vi "StartProcess.vi"(7 "型号":enum16{"长安", "江淮"}(ring), 8 "error in":errorcluster caption="错误输入（无错误）", 9 "延时":i32=100, 10 "Cycles":i32=5, 11 "COMIn":refnum<visa-resource-name>) -> (0 "error out":errorcluster caption="错误输出", 1 "连接的字符串":string, 2 "Time":u32, 3 "OK？":bool)   [LabVIEW 2013]
uses:
  <vilib>/Instr/_visa.llb/VISA Flush IO Buffer Mask.ctl
  <vilib>/Instr/_visa.llb/VISA Configure Serial Port (Instr).vi
panel:
  out "数组 2":string[](array[string])
  out "数组":string[](array[string])
  out "读取缓冲区 3":string
  out "字符串 2":string
  out "读取缓冲区 2":string
  out "字符串":string
  in  "CMD":enum16{"启动进程", "退出进程"}(ring)
  out "读取缓冲区":string
  # "长安登录与启动localdata：\n用户名：root\n密码：quectel123\n启动localdata：/data/QuecOpen/local_data\n江淮登录与启动localdata：\n用户名：root\n密码：oelinux_ls123\n启动localdata：/vendor/app/local_data\n启动localdata修改为：/vendor/app/auto_test_main"
  # "延时取100时较为稳定"
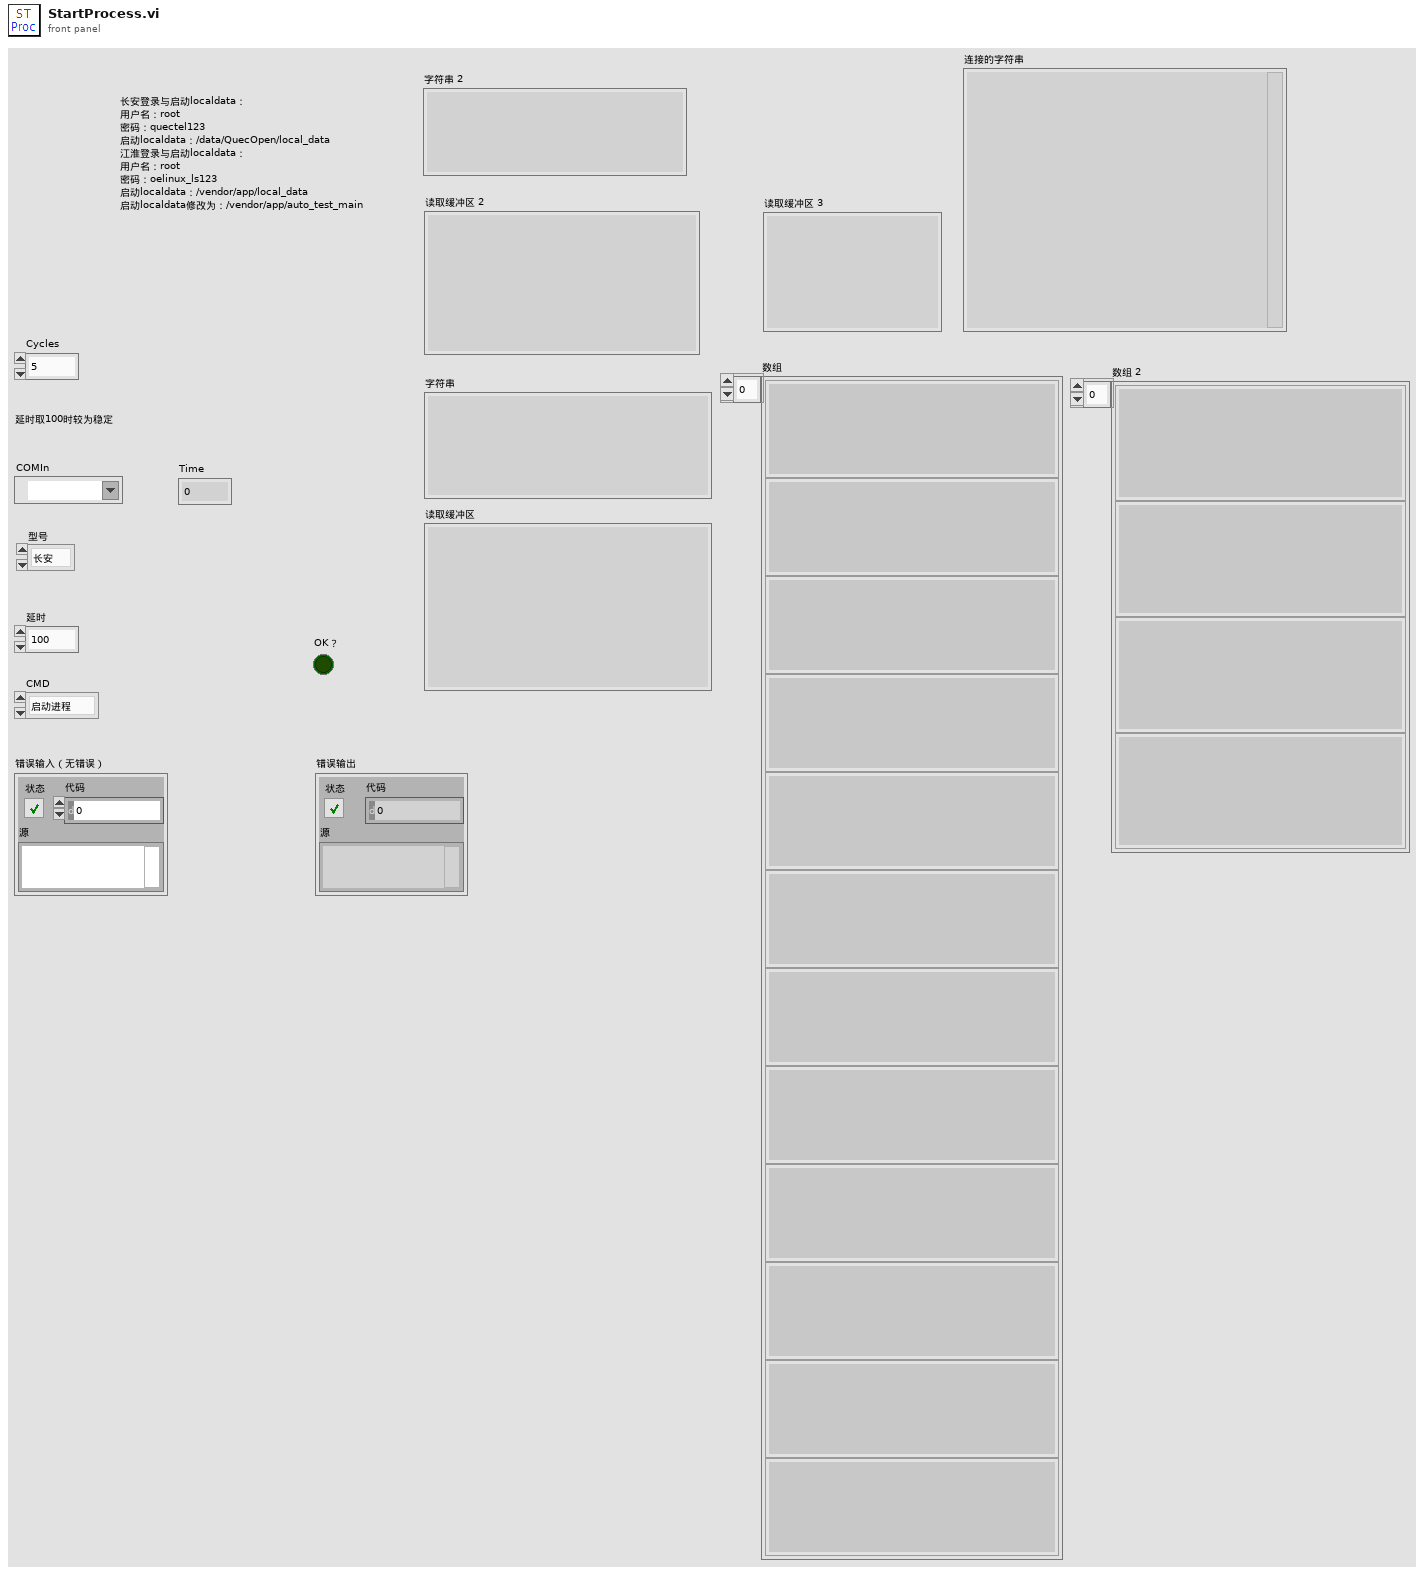
[diagram p1: front panel]
types:
  T1 = typedef "VISA Flush IO Buffer Mask.ctl" = u16
  T2 = cluster{"波特率":u32, "数据比特":u16, "奇偶":enum16{"None", "Odd", "Even", "Mark", "Space"}, "停止位":u16, "流控制":u16}
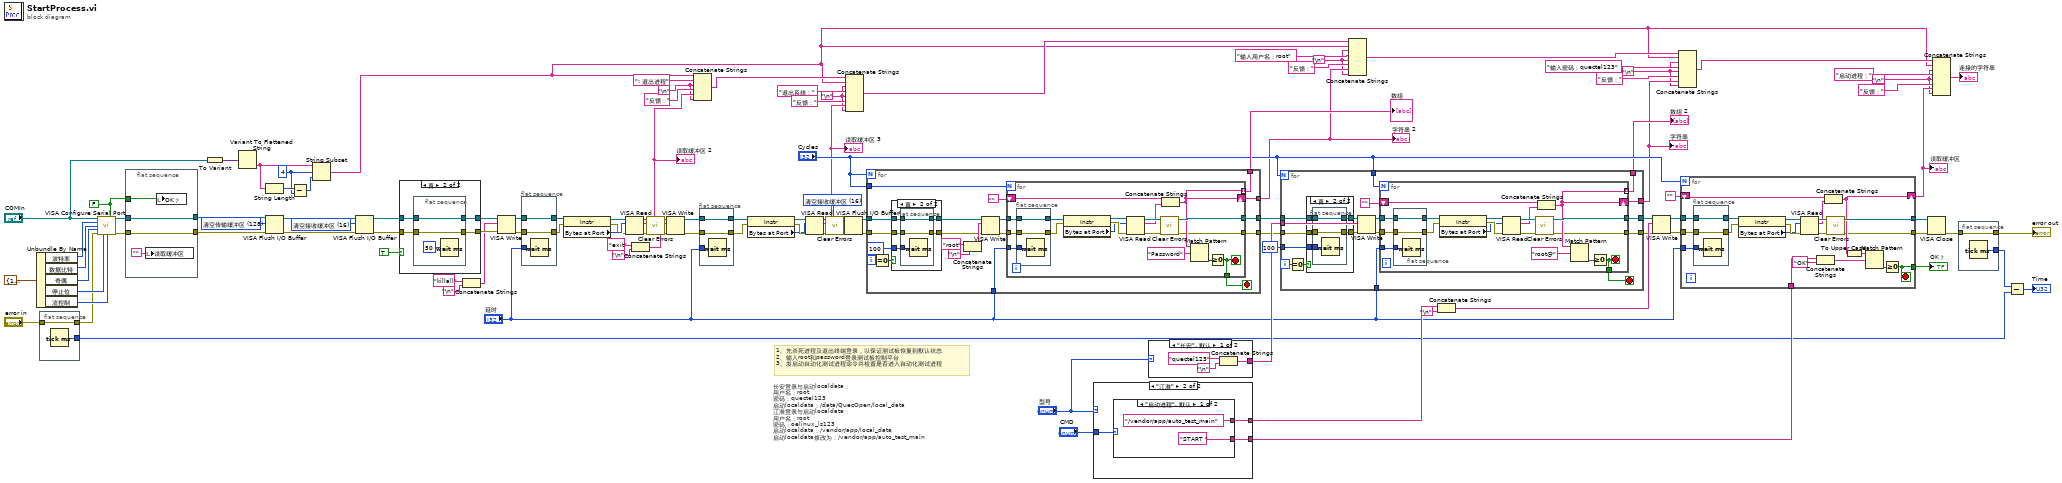
[diagram p0: block diagram]
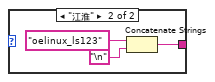
[diagram p2: hidden frame]
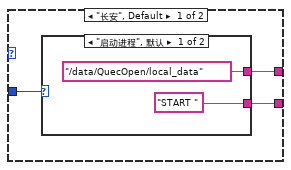
[diagram p3: hidden frame]
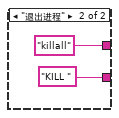
[diagram p4: hidden frame]
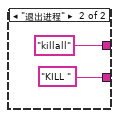
[diagram p5: hidden frame]
diagram:
  w3 = "\n"
  w6 = "\n"
  w8 = "\n"
  w10 = "\n"
  w25 = "\n"
  w31 = 4 ("偏移量(0)")
  w57 = T1 16 items=["清空接收缓冲区"=16, "向设备写入传输缓冲区"=32, "清空接收缓冲区（无I/O）"=64, "清空传输缓冲区"=128] ("Mask")
  w103 = T1 16 items=["清空接收缓冲区"=16, "向设备写入传输缓冲区"=32, "清空接收缓冲区（无I/O）"=64, "清空传输缓冲区"=128] ("Mask")
  w104 = T1 128 items=["清空接收缓冲区"=16, "向设备写入传输缓冲区"=32, "清空接收缓冲区（无I/O）"=64, "清空传输缓冲区"=128] ("Mask")
  w1 = FALSE ("Enable Termination\nChar (T)")
  # "长安登录与启动localdata：\n用户名：root\n密码：quectel123\n启动localdata：/data/QuecOpen/local_data\n江淮登录与启动localdata：\n用户名：root\n密码：oelinux_ls123\n启动localdata：/vendor/app/local_data\n启动localdata修改为：/vendor/app/auto_test_main"
  # "1、先杀死进程及退出终端登录，以保证测试板恢复到默认状态\n2、输入root和password登录测试板控制平台\n3、发启动自动化测试进程命令并检查是否进入自动化测试进程"
  n1 = Unbundle By Name(T2 {"波特率"=115200, "数据比特"=8, "奇偶"=enum."None", "停止位"=10, "流控制"=0} ("串口设置")) -> ("波特率"=w109:u32, "数据比特"=w108:u16, "奇偶"=w107:enum16{"None", "Odd", "Even", "Mark", "Space"}, "停止位"=w106:u16, "流控制"=w105:u16)
  n2 = flat-sequence {
    tunnel: [w112] -> w47
    tunnel: "error in" -> [w112]
    tunnel: [w111] -> w42
    frame #0 {
      n3 = Tick Count (ms)() -> (millisecond timer value=w111:u32)
    }
  }
  n4 = call-poly "VISA Configure Serial Port"("VISA resource name"="COMIn", "Enable Termination\nChar (T)"=w1, "baud rate (9600)"=w109, "data bits (8)"=w108, "parity (0:none)"=w107, "error in (no error)"=w47, "stop bits (10: 1 bit)"=w106, "flow control (0:none)"=w105) -> ("VISA resource name out"=w91:refnum<visa-resource-name>, "error out"=w92:errorcluster)  [unwired: 6 in]
  n5 = flat-sequence {
    tunnel: [w116] -> w93
    tunnel: w92 -> [w116]
    tunnel: [w114] -> w90
    tunnel: w91 -> [w114]
    tunnel: w1 -> [w113]
    frame #0 {
      n6 = local write "读取缓冲区"("") -> ()
      n7 = local write "OK？"(w113) -> ()
    }
  }
  n8 = To Variant(anything="COMIn") -> (Variant=w34:variant)
  n9 = Variant To Flattened String(Variant=w34) -> (data string=w33:string)  [unwired: 1 out]
  n10 = String Length(string=w33) -> (length=w32:i32)
  n11 = VISA Flush I/O Buffer(VISA resource name=w90, mask (16)=w104, error in (no error)=w93) -> (VISA resource name out=w102:refnum<visa-resource-name>, error out=w101:errorcluster)
  n12 = Subtract(x=w32, y=w31) -> (x-y=w30:i32)
  n13 = String Subset(string=w33, offset (0)=w31, length (rest)=w30) -> (substring=w4:string)
  n14 = VISA Flush I/O Buffer(VISA resource name=w102, mask (16)=w103, error in (no error)=w101) -> (VISA resource name out=w100:refnum<visa-resource-name>, error out=w99:errorcluster)
  n15 = case shown="真" TRUE {
    tunnel: w100 -> [w118 w122]
    tunnel: w99 -> [w117 w119]
    tunnel: [w118 w121] -> w82
    tunnel: [w117 w120] -> w81
    frame False {
    }
    frame True {
      n16 = flat-sequence {
        tunnel: [w124] -> w121
        tunnel: w122 -> [w124]
        tunnel: [w123] -> w120
        tunnel: w119 -> [w123]
        frame #0 {
          n17 = Wait (ms)(milliseconds to wait=u32 50 ("毫秒倍数")) -> ()  [unwired: 1 out]
        }
      }
    }
  }
  n18 = Concatenate Strings("killall" ("CMD 2"), "\n") -> (w78:string)
  n19 = VISA Write(VISA resource name=w82, write buffer=w78, error in (no error)=w81) -> (VISA resource name out=w83:refnum<visa-resource-name>, error out=w84:errorcluster)  [unwired: 1 out]
  n20 = flat-sequence {
    tunnel: [w128] -> w85
    tunnel: w83 -> [w128]
    tunnel: [w127] -> w86
    tunnel: w84 -> [w127]
    tunnel: "延时" -> [w126]
    frame #0 {
      n21 = Wait (ms)(milliseconds to wait=w126) -> ()  [unwired: 1 out]
    }
  }
  n22 = property class="Instr"(reference=w85, error in=w86) -> (reference out=w89:refnum<visa-resource-name>, error out=w87:errorcluster, "Bytes at Port"=w88:u32)
  n23 = VISA Read(VISA resource name=w89, byte count=w88, error in (no error)=w87) -> (VISA resource name out=w67:refnum<visa-resource-name>, read buffer=w26:string, error out=w66:errorcluster)  [unwired: 1 out]
  "读取缓冲区 2" <- w26
  n24 = Concatenate Strings("exit" ("CMD 2"), "\n") -> (w63:string)
  n25 = call <vilib>:"Clear Errors.vi"("error in (no error)"=w66) -> ("error out"=w36:errorcluster)  [unwired: 6 in]
  n26 = VISA Write(VISA resource name=w67, write buffer=w63, error in (no error)=w36) -> (VISA resource name out=w62:refnum<visa-resource-name>, error out=w61:errorcluster)  [unwired: 1 out]
  n27 = Concatenate Strings(w4, ": 退出进程", w25, "反馈：", w26, w25) -> (w11:string)
  n28 = flat-sequence {
    tunnel: [w131] -> w53
    tunnel: w62 -> [w131]
    tunnel: [w130] -> w52
    tunnel: w61 -> [w130]
    tunnel: "延时" -> [w129]
    frame #0 {
      n29 = Wait (ms)(milliseconds to wait=w129) -> ()  [unwired: 1 out]
    }
  }
  n30 = property class="Instr"(reference=w53, error in=w52) -> (reference out=w54:refnum<visa-resource-name>, error out=w56:errorcluster, "Bytes at Port"=w55:u32)
  n31 = VISA Read(VISA resource name=w54, byte count=w55, error in (no error)=w56) -> (VISA resource name out=w51:refnum<visa-resource-name>, read buffer=w22:string, error out=w50:errorcluster)  [unwired: 1 out]
  "读取缓冲区 3" <- w22
  n32 = call <vilib>:"Clear Errors.vi"("error in (no error)"=w50) -> ("error out"=w35:errorcluster)  [unwired: 6 in]
  n33 = VISA Flush I/O Buffer(VISA resource name=w51, mask (16)=w57, error in (no error)=w35) -> (VISA resource name out=w59:refnum<visa-resource-name>, error out=w58:errorcluster)
  n34 = Concatenate Strings(w11, w4, w10, "退出系统：", w10, "反馈：", w22, w10) -> (w9:string)
  n35 = for {
    N: "Cycles" -> [_]
    tunnel: [w146] -> w71
    tunnel: [w145] -> w40
    tunnel: w59 -> [w139]
    tunnel: w58 -> [w138]
    tunnel: "延时" -> [w132]
    tunnel: "Cycles" -> [w142]
    tunnel: [w141] -> w19
    tunnel: [w135] -> w49
    i -> [w134]
    stop <- w143 stop-if-true
    n36 = Equal To 0?(x=w134) -> (x = 0?=w133:bool)
    n37 = case shown="真" w133 {
      tunnel: [w153 w158] -> w140
      tunnel: w139 -> [w153 w157]
      tunnel: w138 -> [w152 w156]
      tunnel: [w152 w155] -> w137
      tunnel: 100 -> [_ w154]
      frame False {
      }
      frame True {
        n38 = flat-sequence {
          tunnel: [w161] -> w158
          tunnel: w157 -> [w161]
          tunnel: [w160] -> w155
          tunnel: w156 -> [w160]
          tunnel: [w159] -> _
          tunnel: w154 -> [w159]
          frame #0 {
            n39 = Wait (ms)(milliseconds to wait=w159) -> ()  [unwired: 1 out]
          }
        }
      }
    }
    n40 = Concatenate Strings("root", "\n") -> (w148:string)
    n41 = VISA Write(VISA resource name=w140, write buffer=w148, error in (no error)=w137) -> (VISA resource name out=w147:refnum<visa-resource-name>, error out=w151:errorcluster)  [unwired: 1 out]
    n42 = for {
      N: w142 -> [_]
      tunnel: w151 -> [w178]
      tunnel: w147 -> [w177]
      tunnel: [w176] -> w146
      tunnel: [w162] -> w145
      tunnel: w132 -> [w166]
      shift-right: [w163] -> w141
      shift-left: "" -> [w165]
      tunnel: [w164] -> w143
      tunnel: [w163] -> w135 mode=indexing
      stop <- w164 stop-if-true
      n43 = flat-sequence {
        tunnel: [w181] -> w174
        tunnel: w177 -> [w181]
        tunnel: [w180] -> w173
        tunnel: w178 -> [w180]
        tunnel: w166 -> [w179]
        frame #0 {
          n44 = Wait (ms)(milliseconds to wait=w179) -> ()  [unwired: 1 out]
        }
      }
      n45 = property class="Instr"(reference=w174, error in=w173) -> (reference out=w170:refnum<visa-resource-name>, error out=w172:errorcluster, "Bytes at Port"=w171:u32)
      n46 = VISA Read(VISA resource name=w170, byte count=w171, error in (no error)=w172) -> (VISA resource name out=w176:refnum<visa-resource-name>, read buffer=w169:string, error out=w175:errorcluster)  [unwired: 1 out]
      n47 = call <vilib>:"Clear Errors.vi"("error in (no error)"=w175) -> ("error out"=w162:errorcluster)  [unwired: 6 in]
      n48 = Concatenate Strings(w165, w169) -> (w163:string)
      n49 = Match Pattern(string=w163, regular expression="Password") -> (offset past match=w168:i32)  [unwired: 1 in, 3 out]
      n50 = Greater Or Equal To 0?(x=w168) -> (x >= 0?=w164:bool)
    }
  }
  "字符串 2" <- w19
  "数组" <- w49
  n51 = case shown="\"江淮\"" "型号" {
    tunnel: "CMD" -> [w184 w191]
    tunnel: [w183 w190] -> w73
    tunnel: [w182 w189] -> w72
    frame "长安", Default {
      n52 = case shown="\"启动进程\", 默认" w184 {
        tunnel: ["/data/QuecOpen/local_data" ("CMD 2") "killall" ("CMD 2")] -> w183
        tunnel: ["START " ("CMD 2") "KILL " ("CMD 2")] -> w182
        frame "启动进程", Default {
        }
        frame "退出进程" {
        }
      }
    }
    frame "江淮" {
      n53 = case shown="\"启动进程\", 默认" w191 {
        tunnel: ["/vendor/app/auto_test_main" ("CMD 2") "killall" ("CMD 2")] -> w190
        tunnel: ["START " ("CMD 2") "KILL " ("CMD 2")] -> w189
        frame "启动进程", Default {
        }
        frame "退出进程" {
        }
      }
    }
  }
  n54 = case shown="\"长安\", 默认" "型号" {
    tunnel: [w196 w199] -> w70
    frame "长安", Default {
      n55 = Concatenate Strings("quectel123", "\n") -> (w196:string)
    }
    frame "江淮" {
      n56 = Concatenate Strings("oelinux_ls123", "\n") -> (w199:string)
    }
  }
  n57 = for {
    N: "Cycles" -> [_]
    tunnel: w71 -> [w209]
    tunnel: w70 -> [w219]
    tunnel: [w217] -> w69
    tunnel: [w215] -> w68
    tunnel: [w214] -> w16
    tunnel: "延时" -> [w213]
    tunnel: "Cycles" -> [w211]
    tunnel: w40 -> [w207]
    tunnel: 100 -> [w205]
    tunnel: [w204] -> w37
    i -> [w203]
    stop <- w210 stop-if-true
    n58 = Equal To 0?(x=w203) -> (x = 0?=w202:bool)
    n59 = case shown="真" w202 {
      tunnel: w209 -> [w221 w226]
      tunnel: [w221 w225] -> w208
      tunnel: w207 -> [w220 w224]
      tunnel: [w220 w223] -> w206
      tunnel: w205 -> [_ w222]
      frame False {
      }
      frame True {
        n60 = flat-sequence {
          tunnel: [w229] -> w225
          tunnel: w226 -> [w229]
          tunnel: [w228] -> w223
          tunnel: w224 -> [w228]
          tunnel: [w227] -> _
          tunnel: w222 -> [w227]
          frame #0 {
            n61 = Wait (ms)(milliseconds to wait=w227) -> ()  [unwired: 1 out]
          }
        }
      }
    }
    n62 = VISA Write(VISA resource name=w208, write buffer=w219, error in (no error)=w206) -> (VISA resource name out=w218:refnum<visa-resource-name>, error out=w216:errorcluster)  [unwired: 1 out]
    n63 = for {
      N: w211 -> [_]
      tunnel: w216 -> [w246]
      tunnel: w213 -> [w245]
      tunnel: w218 -> [w244]
      tunnel: [w238] -> w217
      tunnel: [w230] -> w215
      shift-right: [w231] -> w214
      shift-left: "" -> [w236]
      tunnel: [w232] -> w210
      tunnel: [w231] -> w204 mode=indexing
      stop <- w232 stop-if-true
      n64 = flat-sequence {
        tunnel: [w249] -> w243
        tunnel: w244 -> [w249]
        tunnel: [w248] -> w242
        tunnel: w246 -> [w248]
        tunnel: w245 -> [w247]
        frame #0 {
          n65 = Wait (ms)(milliseconds to wait=w247) -> ()  [unwired: 1 out]
        }
      }
      n66 = property class="Instr"(reference=w243, error in=w242) -> (reference out=w239:refnum<visa-resource-name>, error out=w241:errorcluster, "Bytes at Port"=w240:u32)
      n67 = VISA Read(VISA resource name=w239, byte count=w240, error in (no error)=w241) -> (VISA resource name out=w238:refnum<visa-resource-name>, read buffer=w235:string, error out=w237:errorcluster)  [unwired: 1 out]
      n68 = call <vilib>:"Clear Errors.vi"("error in (no error)"=w237) -> ("error out"=w230:errorcluster)  [unwired: 6 in]
      n69 = Concatenate Strings(w236, w235) -> (w231:string)
      n70 = Match Pattern(string=w231, regular expression="root@") -> (offset past match=w234:i32)  [unwired: 1 in, 3 out]
      n71 = Greater Or Equal To 0?(x=w234) -> (x >= 0?=w232:bool)
    }
  }
  "字符串" <- w16
  "数组 2" <- w37
  n72 = Concatenate Strings(w9, w4, w8, "输入用户名：root", w8, "反馈：", w19, w8) -> (w7:string)
  n73 = Concatenate Strings(w73, "\n") -> (w76:string)
  n74 = VISA Write(VISA resource name=w69, write buffer=w76, error in (no error)=w68) -> (VISA resource name out=w75:refnum<visa-resource-name>, error out=w74:errorcluster)  [unwired: 1 out]
  n75 = Concatenate Strings(w7, w4, w6, "输入密码：quectel123", w6, "反馈：", w16, w6) -> (w5:string)
  n76 = for {
    N: "Cycles" -> [_]
    tunnel: [w269] -> w97
    tunnel: [w250] -> w96
    tunnel: [w251] -> w95
    tunnel: w75 -> [w267]
    tunnel: w74 -> [w266]
    tunnel: w72 -> [w257]
    tunnel: "延时" -> [w255]
    shift-right: [w252] -> w13
    shift-left: "" -> [w254]
    stop <- w251 stop-if-true
    n77 = flat-sequence {
      tunnel: [w272] -> w265
      tunnel: w267 -> [w272]
      tunnel: [w271] -> w264
      tunnel: w266 -> [w271]
      tunnel: w255 -> [w270]
      frame #0 {
        n78 = Wait (ms)(milliseconds to wait=w270) -> ()  [unwired: 1 out]
      }
    }
    n79 = property class="Instr"(reference=w265, error in=w264) -> (reference out=w261:refnum<visa-resource-name>, error out=w263:errorcluster, "Bytes at Port"=w262:u32)
    n80 = VISA Read(VISA resource name=w261, byte count=w262, error in (no error)=w263) -> (VISA resource name out=w269:refnum<visa-resource-name>, read buffer=w253:string, error out=w268:errorcluster)  [unwired: 1 out]
    n81 = Concatenate Strings(w257, "OK" ("正则表达式")) -> (w256:string)
    n82 = Concatenate Strings(w254, w253) -> (w252:string)
    n83 = call <vilib>:"Clear Errors.vi"("error in (no error)"=w268) -> ("error out"=w250:errorcluster)  [unwired: 6 in]
    n84 = To Upper Case(1:w252) -> (0:w259:string)
    n85 = Match Pattern(string=w259, regular expression=w256) -> (offset past match=w260:i32)  [unwired: 1 in, 3 out]
    n86 = Greater Or Equal To 0?(x=w260) -> (x >= 0?=w251:bool)
  }
  "OK？" <- w95
  "读取缓冲区" <- w13
  n87 = VISA Close(VISA resource name=w97, error in (no error)=w96) -> (error out=w45:errorcluster)
  n88 = Concatenate Strings(w5, w4, w3, "启动进程：", w3, "反馈：", w13, w3) -> (→"连接的字符串":string)
  n89 = flat-sequence {
    tunnel: [w274] -> w44
    tunnel: w45 -> [w274]
    tunnel: [w273] -> w43
    frame #0 {
      n90 = Tick Count (ms)() -> (millisecond timer value=w273:u32)
    }
  }
  n91 = Subtract(x=w43, y=w42) -> (x-y=→"Time":u32)
  "error out" <- w44
